vi "Robot Global Data.vi"() -> ()   [LabVIEW 2012]
doc: "This global VI can contain as many global variables as you need. Place a control on the panel, give it a good name. To read or write to it from a VI, drag the icon to the diagram of that VI. You can also drag from the project. Click on the node to change which global you access. You shouldn't have multiple locations writing to a global or it will cause a race-condition."
uses:
  <vilib>/Rock Robotics/WPI/Camera/WPI_CameraImageSize.ctl
  <vilib>/Rock Robotics/WPI/DriverStation/WPI_DriverStationRobotMode2.ctl
panel:
  in  "Autonomous TARF Voltage":dbl=2.84
  out "IsTeleop":bool
  in  "TARF Pot V2":dbl
  in  "TARF Pot V1":dbl
  in  "Enable Autonomous":bool
  in  "Time To Lower TARF In Autonomous":u32
  out "Climber Arm At Position":bool
  out "TARF Down":bool
  in  "Autonomous Tarf Angle":dbl
  in  "Clamp State":u16
  in  "TeleOp Elapsed Seconds":dbl
  in  "Dump Speed Outside":dbl
  in  "Dump Speed Inside":dbl
  in  "TARF Angle Red":dbl
  in  "TARF Angle Blue":dbl
  in  "State Delay":u32=1000
  out "Climber Button Unlocked":bool=TRUE
  in  "Climber State":u8
  in  "TARF Manual":bool
  in  "Emergency Climber Stop":bool
  in  "Climber Arm Manual":bool
  in  "Soft Stop Min":dbl=0.4
  in  "Soft Stop Max":dbl=39.8
  in  "Climber Arm Tolerance":dbl=0.25
  in  "Desired Climber Arm Position":dbl=29.0
  out "Tail Closed":bool
  in  "Climber Arm Inches Per Volt":dbl
  in  "Actual Climber Arm Position":dbl
  in  "Drive Ramp Constant Y":dbl=0.03
  in  "Drive Mechanical Deadband Y":dbl=0.3
  in  "Drive Mechanical Deadband X":dbl=0.3
  out "TARF At Desired Angle":bool
  in  "TARF Angle Tolerance":dbl=1.0
  in  "Desired TARF Angle":dbl
  in  "Actual TARF Angle":dbl
  in  "Robot Mode":T1
  in  "LED toggle rate (ms)":u32=20
  in  "image size":T2=enum."320x240"
  in  "Enable Vision":bool
  # "deg"
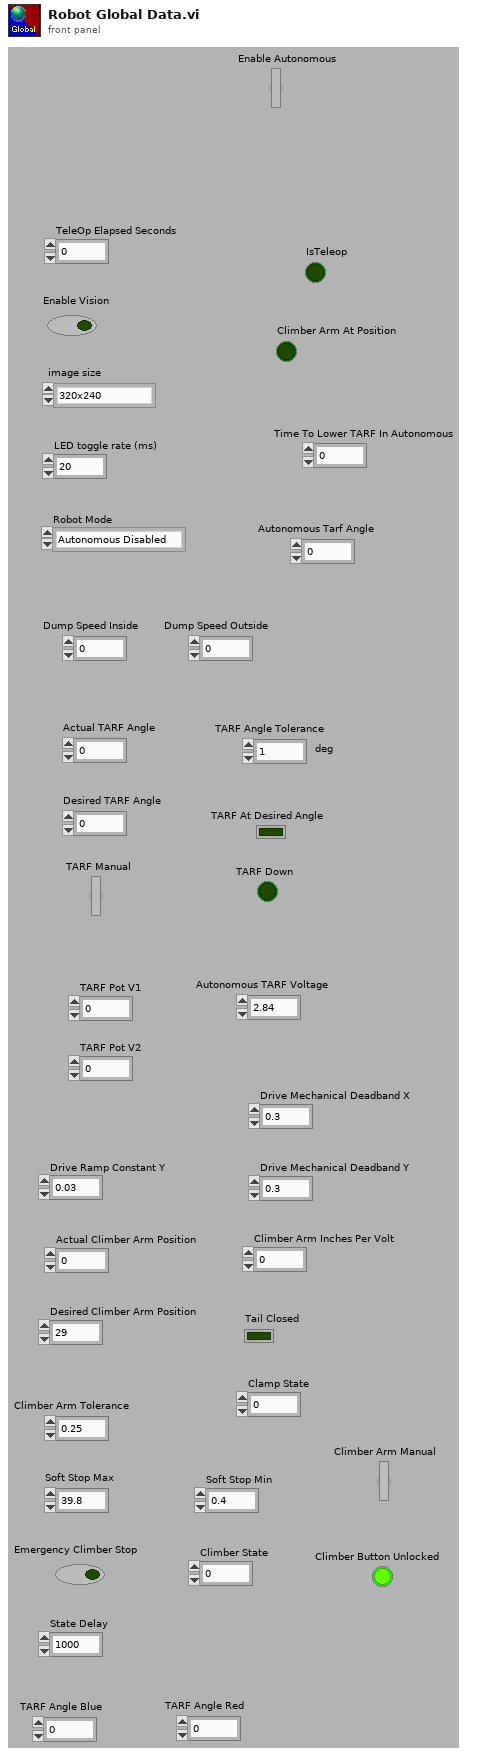
[diagram p1: front panel]
types:
  T1 = typedef "WPI_DriverStationRobotMode2.ctl" = enum16{"Autonomous Disabled", "Autonomous Enabled", "Teleop Disabled", "Teleop Enabled", "Timeout", "Finish", "Test Disabled", "Test Enabled"}
  T2 = typedef "WPI_CameraImageSize.ctl" = enum16{"640x480", "320x240", "160x120"}
diagram:
